vi "logical_series.get.vi"(8 "error in":errorcluster, 11 "Nominal Client in":refnum<class "Nominal Client.lvclass">) -> (0 "error out":errorcluster, 1 "Response Headers":refnum<class "Response Headers.lvclass">, 2 "Response":string, 3 "Nominal Client out":refnum<class "Nominal Client.lvclass">)   [LabVIEW 2020, in "Nominal Client.lvclass"]
doc: "Get a logical series by logical series rid."
uses:
  Nominal Client.lvclass
  <vilib>/addons/_JKI.lib/REST Client/classes/Response Headers/Response Headers.lvclass
  Nominal Client.lvclass/Nominal Client.ctl
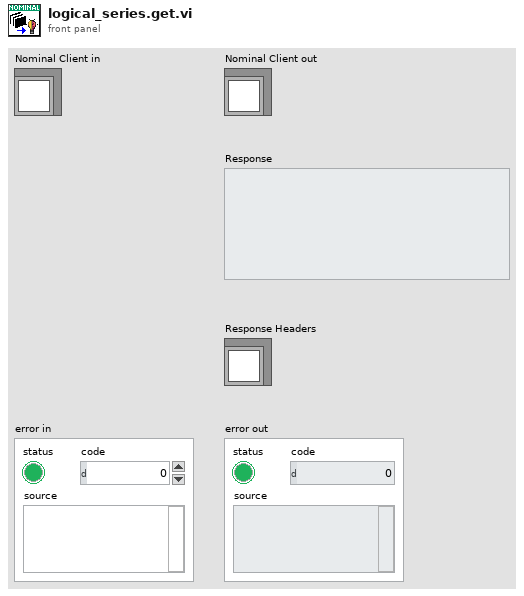
[diagram p1: front panel]
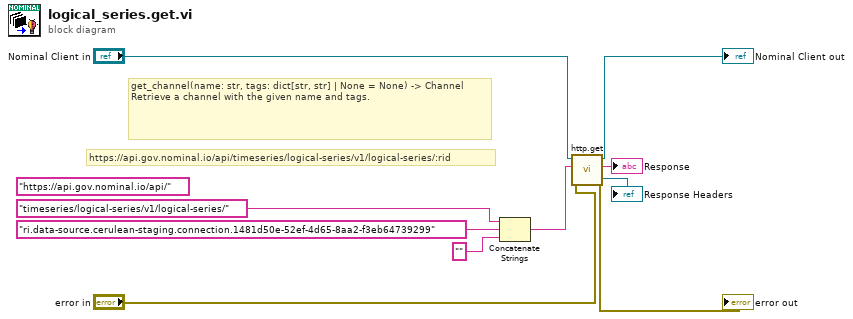
[diagram p0: block diagram]
diagram:
  (unwired) "https://api.gov.nominal.io/api/" ("Base URL")
  # "get_channel(name: str, tags: dict[str, str] | None = None) -> Channel\nRetrieve a channel with the given name and tags."
  # "https://api.gov.nominal.io/api/timeseries/logical-series/v1/logical-series/:rid"
  n1 = Concatenate Strings("timeseries/logical-series/v1/logical-series/" ("Path"), "ri.data-source.cerulean-staging.connection.1481d50e-52ef-4d65-8aa2-f3eb64739299" ("string"), "" ("string")) -> (w9:string)
  n2 = call "http.get.vi"("error in"="error in", "Path"=w9, "Nominal Client in"="Nominal Client in") -> ("error out"=→"error out":errorcluster, "Response"=→"Response":string, "Nominal Client out"=→"Nominal Client out":refnum<class "Nominal Client.lvclass">, "Response Headers"=→"Response Headers":refnum<class "Response Headers.lvclass">)  [unwired: 5 in]
